vi "add_line_to_table.vi"(8 "error in (no error)":errorcluster, 10 "new table line":string[](array[string]), 11 "MagFieldTable in":refnum<class "MagFieldTable.lvclass">) -> (0 "error out":errorcluster, 3 "MagFieldTable out":refnum<class "MagFieldTable.lvclass">)   [LabVIEW 2018, in "MagFieldTable.lvclass"]
uses:
  MagFieldTable.lvclass
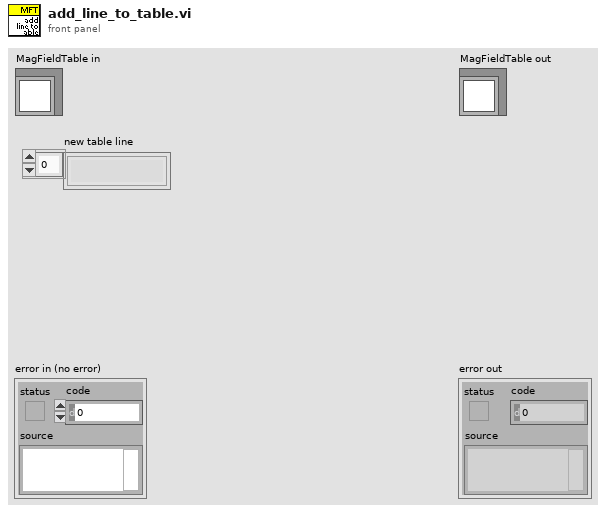
[diagram p1: front panel]
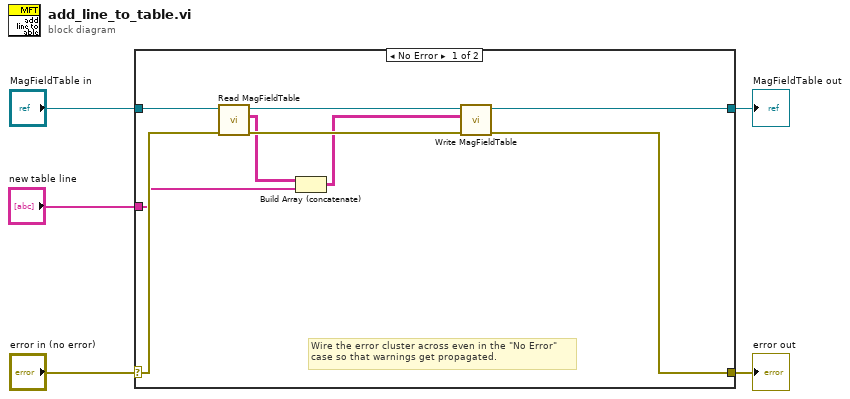
[diagram p0: block diagram]
diagram:
  n1 = case shown="No Error" "error in (no error)" {
    selector: "error in (no error)" -> [w11 w16]
    tunnel: [w9 w16] -> w4
    tunnel: [w12 w15] -> w2
    tunnel: "MagFieldTable in" -> [w14 w15]
    tunnel: "new table line" -> [w7 _]
    frame No Error {
      # "Wire the error cluster across even in the \"No Error\"\ncase so that warnings get propagated."
      n2 = call-dynamic "Read MagFieldTable.vi"("error in (no error)"=w11, "MagFieldTable in"=w14) -> ("error out"=w10:errorcluster, "MagFieldTable"=w8:string[][], "MagFieldTable out"=w13:refnum<class "MagFieldTable.lvclass">)  [unwired: 7 in]
      n3 = Build Array (concatenate)(w8, w7) -> (w6:string[][])
      n4 = call-dynamic "Write MagFieldTable.vi"("error in (no error)"=w10, "MagFieldTable"=w6, "MagFieldTable in"=w13) -> ("error out"=w9:errorcluster, "MagFieldTable out"=w12:refnum<class "MagFieldTable.lvclass">)  [unwired: 7 in]
    }
    frame Error {
    }
  }
  "error out" <- w4
  "MagFieldTable out" <- w2
